vi "CLI.git-flow.vi"(6 "name":string, 8 "error in (no error)":errorcluster, 9 "Branch":T2="feature", 10 "Command":T1="config", 11 "Git in":refnum<class "Git.lvclass">) -> (0 "error out":errorcluster, 1 "standard error":string, 2 "standard output":string, 3 "Git out":refnum<class "Git.lvclass">, 4 "return code":i32)   [LabVIEW 2019, in "Git.lvclass"]
uses:
  Git.lvclass
  Typedefs/Branches.git-flow--combo.ctl
  Typedefs/Commands.git-flow--combo.ctl
  Git.lvclass/Git.ctl
panel:
  # "Fatal: Not a git repository"
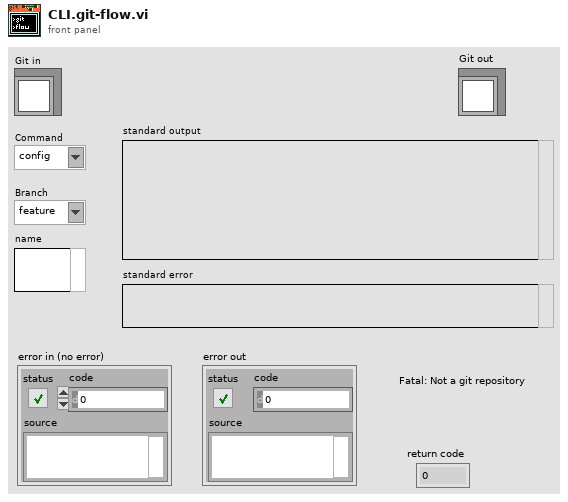
[diagram p1: front panel]
types:
  T1 = typedef "Git.lvclass/Commands.git-flow--combo.ctl" = string
  T2 = typedef "Git.lvclass/Branches.git-flow--combo.ctl" = string
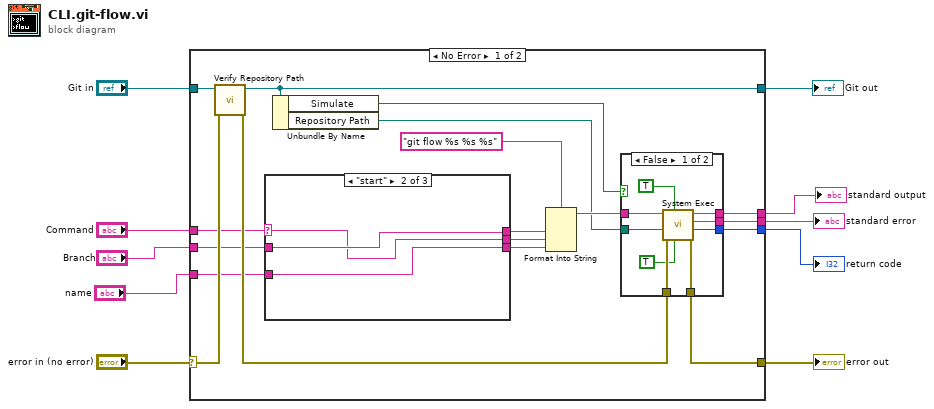
[diagram p0: block diagram]
diagram:
  n1 = case shown="No Error" "error in (no error)" {
    selector: "error in (no error)" -> [w17 w46]
    tunnel: [w28 _] -> w10
    tunnel: [w27 w46] -> w9
    tunnel: "Branch" -> [w13 _]
    tunnel: "Command" -> [w14 _]
    tunnel: [w26 _] -> w6
    tunnel: [w25 _] -> w5
    tunnel: "Git in" -> [w24 w45]
    tunnel: [w22 w45] -> w3
    tunnel: "name" -> [w16 _]
    frame No Error {
      n2 = call "Verify Repository Path.vi"("error in (no error)"=w17, "Git in"=w24) -> ("error out"=w23:errorcluster, "Git out"=w22:refnum<class "Git.lvclass">)  [unwired: 8 in]
      n3 = case shown="\"start\"" w14 {
        selector: w14 -> [w40 w42 w44]
        tunnel: [_ w42 _] -> w15
        tunnel: [w40 w43 w44] -> w21
        tunnel: w16 -> [_ w41 _]
        tunnel: w13 -> [_ w43 _]
        tunnel: [_ w41 _] -> w12
        frame "config", "init", "version" {
        }
        frame "start" {
        }
        frame Default {
        }
      }
      n4 = Unbundle By Name(w22) -> ("Simulate"=w11:bool, "Repository Path"=w18:path)
      n5 = Format Into String(format string="git flow %s %s %s", w21, w15, w12) -> (resulting string=w20:string)  [unwired: 2 in, 1 out]
      n6 = case shown="False" w11 {
        tunnel: [w37 w39] -> w28
        tunnel: [w36 w38] -> w27
        tunnel: [w35 _] -> w26
        tunnel: [w34 _] -> w25
        tunnel: w23 -> [w33 w38]
        tunnel: w20 -> [w32 w39]
        tunnel: w18 -> [w31 _]
        frame False {
          n7 = call <vilib>:"System Exec.vi"("run minimized? (F)"=TRUE, "wait until completion? (T)"=TRUE, "error in (no error)"=w33, "working directory"=w31, "command line"=w32) -> ("error out"=w36:errorcluster, "return code"=w34:i32, "standard error"=w35:string, "standard output"=w37:string)  [unwired: 3 in]
        }
        frame True {
        }
      }
    }
    frame Error {
    }
  }
  "standard output" <- w10
  "standard error" <- w6
  "return code" <- w5
  "error out" <- w9
  "Git out" <- w3
